vi "Configure VI Analzyer.vi"(8 "error in (no error)":errorcluster, 10 "JSON String":string) -> (0 "error out":errorcluster, 3 "VI Analyzer out":refnum<class "VI Analyzer.lvclass">)   [LabVIEW 2014, in "VI Analyzer.lvclass"]
uses:
  VI Analyzer.lvclass
  VI Analyzer - STYP.ctl
  Classes/Job/Job.lvclass/Job.ctl
  VI Analyzer.lvclass/VI Analyzer.ctl
  Classes/Job/Job.lvclass
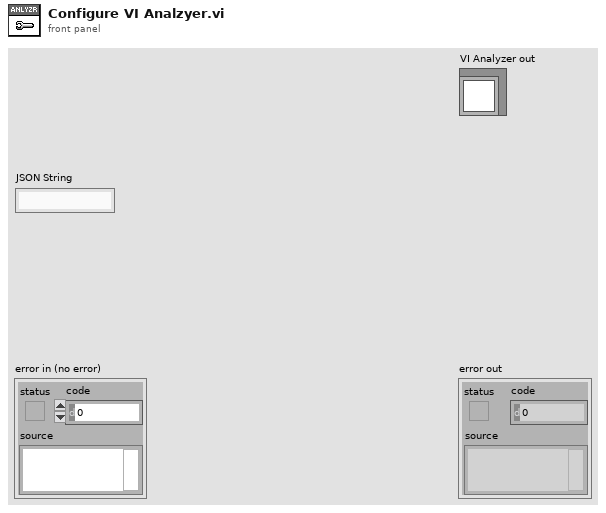
[diagram p1: front panel]
types:
  T1 = typedef "VI Analyzer - STYP.ctl" = cluster{"Executor_Number":string, "Workspace_Path":string, "Test File":string}
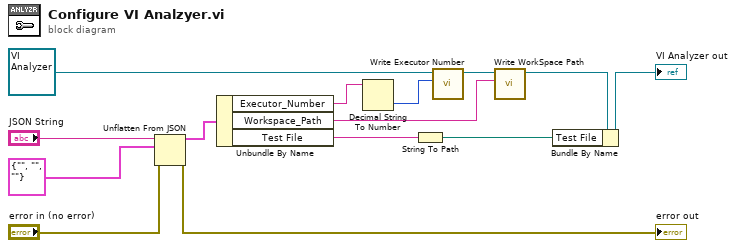
[diagram p0: block diagram]
diagram:
  n1 = Unflatten From JSON(JSON string="JSON String", type and defaults=T1 {"Executor_Number"="", "Workspace_Path"="", "Test File"=""} ("VI Analyzer - STYP.ctl"), error in (no error)="error in (no error)") -> (value=w11:T1, error out=→"error out":errorcluster)  [unwired: 4 in]
  n2 = Unbundle By Name(w11) -> ("Executor_Number"=w10:string, "Workspace_Path"=w6:string, "Test File"=w4:string)
  n3 = Decimal String To Number(string=w10) -> (number=w7:i32)  [unwired: 2 in, 1 out]
  n4 = String To Path(string=w4) -> (path=w3:path)
  n5 = call "Write Executor Number.vi"("Executor Number"=w7, "Job in"=refnum<class "VI Analyzer.lvclass"> refnum ("VI Analyzer in")) -> ("Job out"=w8:refnum<class "VI Analyzer.lvclass">)  [unwired: 8 in, 1 out]
  n6 = call "Write WorkSpace Path.vi"("WorkSpace Path"=w6, "Job in"=w8) -> ("Job out"=w5:refnum<class "VI Analyzer.lvclass">)  [unwired: 8 in, 1 out]
  n7 = Bundle By Name(cluster=w5, "Test File"=w3) -> (→"VI Analyzer out":refnum<class "VI Analyzer.lvclass">)
